vi "Regler Durchfluss LP.vi"(7 "Index":i32, 8 "Fehler":errorcluster caption="Fehler (Eingang)") -> (0 "Fehler (Ausgang)":errorcluster)   [LabVIEW 2020, in "Regler.lvlib" / "Druckregler.lvlib"]
uses:
  Druckregler.lvlib
  Aktionen Param. Druckregler.ctl
  Aktionen Interne Werte.ctl
  Verwaltung/FGV IN Aktionen.ctl
  Allgemein/Aktion FGV Messbetrieb.ctl
  Allgemein/FGV Zustaende Aktionen.ctl
  Allgemein/Aktion FGV T90.ctl
  Allgemein/Aktionen FGV Dichtheitstest.ctl
  Konfig-Dateien/FGV Betriebsdaten Aktionen.ctl
  Verwaltung/Verwaltung - cRIO.lvlib
  Konfig-Dateien/Konfig-Dateien.lvlib
  Regler.lvlib
  Aktion FGV Werte vorgeben.ctl
  Allgemein/Allgemein.lvlib
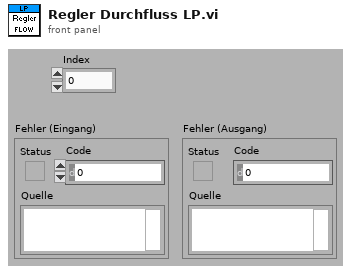
[diagram p1: front panel]
types:
  T1 = typedef "Allgemein.lvlib/Aktionen FGV Dichtheitstest.ctl" = enum16{"lesen", "schreiben"}
  T2 = typedef "Allgemein.lvlib/Aktion FGV T90.ctl" = enum16{"lesen", "schreiben"}
  T3 = typedef "Allgemein.lvlib/FGV Zustaende Aktionen.ctl" = enum16{"lesen", "Zustand PC", "Zustand cRIO", "Bildnummer", "Samplepoint", "Sysloglevel"}
  T4 = typedef "Allgemein.lvlib/Aktion FGV Messbetrieb.ctl" = enum16{"lesen", "schreiben"}
  T5 = typedef "Verwaltung - cRIO.lvlib/FGV IN Aktionen.ctl" = enum16{"lesen", "DI", "AI", "Fühler Br.", "TC", "Fühler Br. TC"}
  T6 = typedef "Regler.lvlib/Druckregler.lvlib/Aktionen Interne Werte.ctl" = enum16{"lesen", "FT-IR", "Ausgang", "Pumpe", "laden", "speichern", "Änderung?", "Druck Kalter Block", "Dichtheitstest"}
  T7 = typedef "Regler.lvlib/Druckregler.lvlib/Aktionen Param. Druckregler.ctl" = enum16{"lesen", "schreiben", "Regler FT-IR", "Regler Ausgang", "Regler Durchfluss", "Regler PMA", "Regler NDIR", "Regler Filterblock", "Regler Gaskühler", "Regler Kalter Block"}
  T8 = typedef "Funktionstasten.lvlib/Zustaende.ctl" = enum16{"Standby", "Pause", "Eco", "Messen", "Kalibrieren", "Spülen Filter", "Spülen Leitung", "Umgebungsluft", "0-Gas", "Cal-Gas", "CG zu PNS", "-------------", "Init 1", "Init 2", "Init 3", "Init 4", "Messen vorbereiten", "Messen durchführen", "Exit"}
  T9 = typedef "Konfig-Dateien.lvlib/FGV Betriebsdaten Aktionen.ctl" = enum16{"lesen", "Anlagengrenzw.", "PID Param.", "Sonstige", "Sensor Para."}
  T10 = typedef "Anlagengrenzwerte.lvlib/Anlagen-Grenzwerte Anzeige.ctl" = cluster{"Eingangsdruck FT-IR:":T11, "Durchfluss FT-IR:":T11, "Durchfluss CalGas:":T11, "Druck Ausgang:":T11, "Druck Kalter Block:":T11, "Heizleitungen intern:":T11, "Heizleitung zu FT-IR:":T11, "Heizung Filterblock:":T11, "Heizung Pumpe:":T11, "Heizleitung Extern SP1:":T11, "Heizleitung Extern SP2:":T11, "FT-IR Heizung Messzelle:":T11, "Schaltschranktemperatur:":T11, "Gaskühler:":T11}
  T11 = typedef "Anlagengrenzwerte.lvlib/Anlagen-Parameter Anzeige.ctl" = cluster{"Sollwert":sgl, "Warn-Min":sgl, "Warn-Max":sgl, "Abschalt-Min":sgl, "Abschalt-Max":sgl, "Regler":u16}
  T12 = typedef "Verwaltung - cRIO.lvlib/Analog Eingaenge.ctl" = cluster{"AI0: Durchfluss FT-IR":sgl, "AI1: Druck Ausgang":sgl, "AI2: Umgebungsdruck":sgl, "AI3: Druck FT-IR":sgl, "AI4: Druck CalGas":sgl, "AI5: Reserve":sgl, "AI6: Reserve":sgl, "AI7: Reserve":sgl, "Rohwert Durchfluss FT-IR":sgl, "Rohwert Druck Ausgang":sgl, "Rohwert Umgebungsdruck":sgl, "Rohwert Druck FT-IR":sgl, "Rohwert Druck CalGas":sgl, "Rohwert AI5":sgl, "Rohwert AI6":sgl, "Rohwert AI7":sgl, "Rohwert Diffdruck mbar FTIR":sgl}
  T13 = typedef "Regler.lvlib/Aktion FGV Werte vorgeben.ctl" = enum16{"lesen", "P-Flow", "D-Filterblock"}
  T14 = cluster{"Numerisch":sgl, "Numerisch":sgl, "Numerisch":sgl, "Numerisch":sgl, "Numerisch":sgl}
  T15 = typedef "Regler.lvlib/Druckregler.lvlib/Regler Interne Werte.ctl" = cluster{"PV":sgl, "D-action":sgl, "Error":sgl, "I-action":sgl, "OUT":sgl}
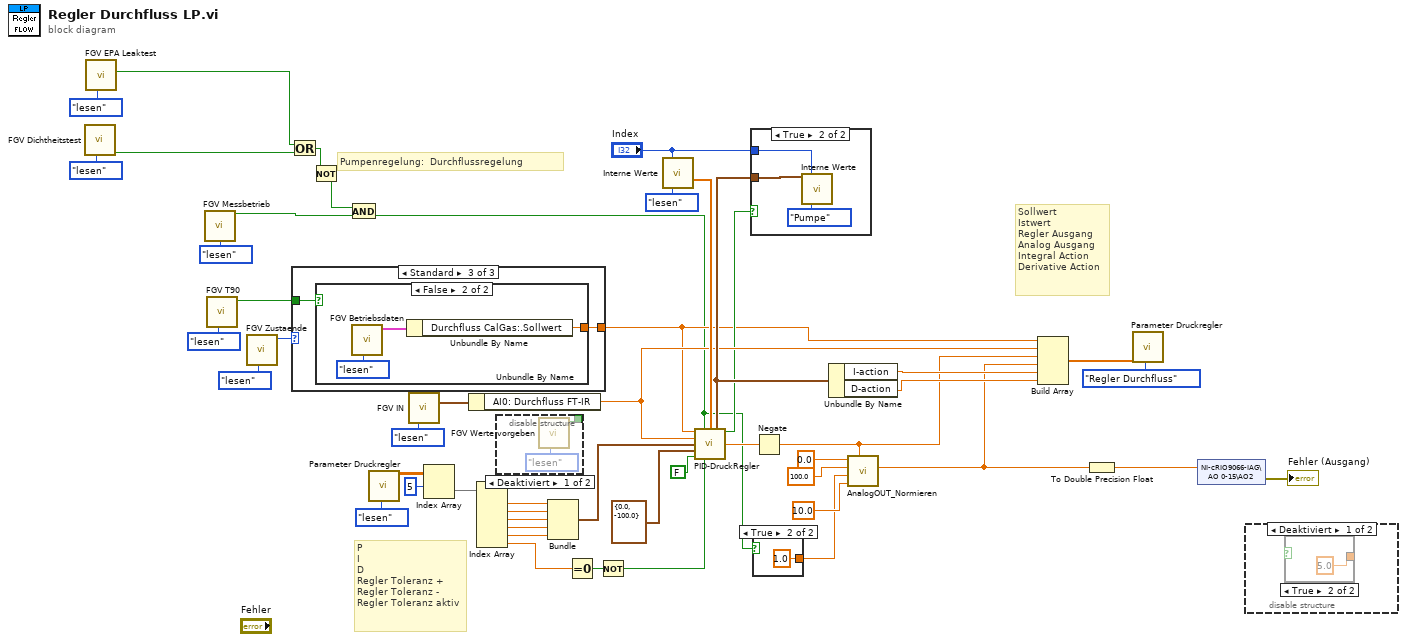
[diagram p0: block diagram]
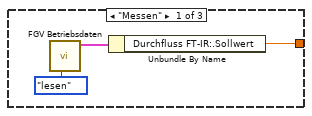
[diagram p2: hidden frame]
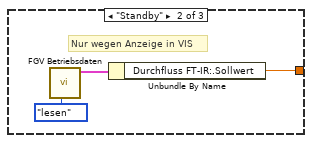
[diagram p3: hidden frame]
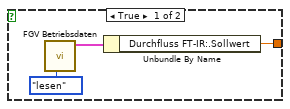
[diagram p4: hidden frame]
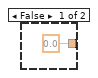
[diagram p6: hidden frame]
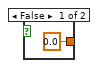
[diagram p9: hidden frame]
diagram:
  # "Pumpenregelung:  Durchflussregelung"
  # "Sollwert\nIstwert\nRegler Ausgang\nAnalog Ausgang\nIntegral Action\nDerivative Action"
  # "P\nI\nD\nRegler Toleranz +\nRegler Toleranz -\nRegler Toleranz aktiv"
  n1 = call "FGV Dichtheitstest.vi"("Aktionen"=Aktionen_FGV_Dichtheitstest."lesen") -> ("Dichtheitstest?"=w6:bool)  [unwired: 9 in, 1 out]
  n2 = call "FGV EPA Leaktest.vi"("Aktion"=enum16{"lesen", "schreiben"}."lesen") -> ("Leaktest aktiv"=w4:bool)  [unwired: 9 in, 1 out]
  n3 = call "FGV Messbetrieb.vi"("Aktion"=Aktion_FGV_Messbetrieb."lesen") -> ("messen"=w12:bool)  [unwired: 13 in, 1 out]
  n4 = call "FGV T90.vi"("Aktion"=Aktion_FGV_T90."lesen") -> ("T90 aktiv"=w8:bool)  [unwired: 7 in, 3 out]
  n5 = call "FGV Zustaende.vi"("Aktionen"=FGV_Zustaende_Aktionen."lesen") -> ("Zustand PC"=w10:T8)  [unwired: 6 in, 4 out]
  n6 = Or(x=w4, y=w6) -> (x .or. y?=w2:bool)
  n7 = case shown="Standard" w10 {
    tunnel: [w51 w54 w58] -> w18
    tunnel: w8 -> [_ _ w57]
    frame "Messen" {
      n8 = call "FGV Betriebsdaten.vi"("Aktionen"=FGV_Betriebsdaten_Aktionen."lesen") -> ("Anlagen-Grenzwerte"=w52:T10)  [unwired: 7 in, 3 out]
      n9 = Unbundle By Name(w52) -> ("Durchfluss FT-IR:.Sollwert"=w51:sgl)
    }
    frame "Standby" {
      # "Nur wegen Anzeige in VIS"
      n10 = call "FGV Betriebsdaten.vi"("Aktionen"=FGV_Betriebsdaten_Aktionen."lesen") -> ("Anlagen-Grenzwerte"=w55:T10)  [unwired: 7 in, 3 out]
      n11 = Unbundle By Name(w55) -> ("Durchfluss FT-IR:.Sollwert"=w54:sgl)
    }
    frame Default {
      n12 = case shown="False" w57 {
        tunnel: [w61 w64] -> w58
        frame True {
          n13 = call "FGV Betriebsdaten.vi"("Aktionen"=FGV_Betriebsdaten_Aktionen."lesen") -> ("Anlagen-Grenzwerte"=w59:T10)  [unwired: 7 in, 3 out]
          n14 = Unbundle By Name(w59) -> ("Durchfluss FT-IR:.Sollwert"=w61:sgl)
        }
        frame False {
          n15 = call "FGV Betriebsdaten.vi"("Aktionen"=FGV_Betriebsdaten_Aktionen."lesen") -> ("Anlagen-Grenzwerte"=w62:T10)  [unwired: 7 in, 3 out]
          n16 = Unbundle By Name(w62) -> ("Durchfluss CalGas:.Sollwert"=w64:sgl)
        }
      }
    }
  }
  n17 = Not(x=w2) -> (.not. x?=w1:bool)
  n18 = And(x=w1, y=w12) -> (x .and. y?=w3:bool)
  n19 = call "Parameter Druckregler.vi"("Aktionen"=Aktionen_Param._Druckregler."lesen") -> ("Regleparameter"=w30:sgl[][])  [unwired: 10 in, 8 out]
  n20 = call "FGV IN.vi"("Aktion"=FGV_IN_Aktionen."lesen") -> ("Analog Eingänge"=w19:T12)  [unwired: 10 in, 4 out]
  n21 = Index Array(array=w30, index (row)=5 ("Index (Zeile)")) -> (element=w29:sgl[])  [unwired: 1 in]
  n22 = Unbundle By Name(w19) -> ("AI0: Durchfluss FT-IR"=w31:sgl)
  n23 = Index Array(array=w29) -> (element #1=w40:sgl, element #2=w39:sgl, element #3=w38:sgl, element #4=w37:sgl, element #5=w36:sgl, element #6=w27:sgl)  [unwired: 6 in]
  n24 = disable-structure shown="Deaktiviert" {
    disable-tunnel: [w65 _] -> _
    frame Disabled {
      n25 = call "FGV Werte vorgeben.vi"("Aktion"=Aktion_FGV_Werte_vorgeben."lesen") -> ("P-Flow"=w65:bool)  [unwired: 9 in, 1 out]
    }
    frame Enabled {
    }
  }
  n26 = Bundle("Numerisch"=w40, "Numerisch"=w39, "Numerisch"=w38, "Numerisch"=w37, "Numerisch"=w36) -> (w35:T14)  [unwired: 1 in]
  n27 = Equal To 0?(x=w27) -> (x = 0?=w34:bool)
  n28 = Not(x=w34) -> (.not. x?=w33:bool)
  n29 = call "Interne Werte.vi"("Index"="Index", "Aktionen Interne Werte"=Aktionen_Interne_Werte."lesen") -> ("Pumpe"=w46:sgl[])  [unwired: 7 in, 6 out]
  n30 = call "PID-DruckRegler.vi"("Sollwert"=w18, "Regler EIN"=w3, "Regler Interne Werte"=w46, "Istwert"=w31, "PID-Parameter"=w35, "output range"=cluster{"output high":sgl, "output low":sgl} {"output high"=0.0, "output low"=-100.0}, "Dichtheitstest"=FALSE, "Regler Toleranz verwenden?"=w33) -> ("Regler Interne Werte"=w45:T15, "Interne Werte speichern"=w23:bool, "Output"=w26:sgl)  [unwired: 5 in]
  n31 = case shown="True" w23 {
    tunnel: "Index" -> [_ w68]
    tunnel: w45 -> [_ w67]
    frame False {
    }
    frame True {
      n32 = call "Interne Werte.vi"("Regler Interne Werte"=w67, "Index"=w68, "Aktionen Interne Werte"=Aktionen_Interne_Werte."Pumpe") -> ()  [unwired: 6 in, 7 out]
    }
  }
  n33 = case shown="True" w3 {
    tunnel: [sgl 0.0 ("Untergrenze") sgl 1.0 ("Untergrenze")] -> w15
    frame False {
    }
    frame True {
    }
  }
  n34 = Negate(x=w26) -> (-x=w16:sgl)
  n35 = Unbundle By Name(w45) -> ("I-action"=w21:sgl, "D-action"=w22:sgl)
  n36 = call "AnalogOUT_Normieren.vi"("Analogwert"=w16, "Obergrenze"=sgl 10.0, "Untergrenze"=w15, "Max Analogwert"=sgl 100.0, "Min Analogwert"=sgl 0.0) -> ("Normierter Wert"=w17:sgl)  [unwired: 6 in]
  n37 = Build Array(w18, w31, w16, w17, w21, w22) -> (w49:sgl[])
  n38 = To Double Precision Float(number=w17) -> (double precision float=w48:dbl)
  n39 = call "Parameter Druckregler.vi"("Werte Durchfluss"=w49, "Aktionen"=Aktionen_Param._Druckregler."Regler Durchfluss") -> ()  [unwired: 9 in, 9 out]
  n40 = shared-variable "NI-cRIO9066-IAG\\AO 0-15\\AO2"(w48) -> (error out=→"Fehler (Ausgang)":errorcluster)  [unwired: 1 in]
  n41 = disable-structure shown="Deaktiviert" {
    frame Disabled {
      n42 = case shown="True" {
        selector: _ -> [_ _]
        tunnel: [sgl 0.0 ("f") sgl 5.0 ("f")] -> _
        frame False {
        }
        frame True {
        }
      }
    }
    frame Enabled {
    }
  }
